vi "Filter VISA COM.vi"(8 "Error In":errorcluster, 11 "Names in":string[](array[string])) -> (0 "Error Out":errorcluster, 2 "Original list":string[](array[string]), 3 "COM only list":string[](array[string]))   [LabVIEW 2018]
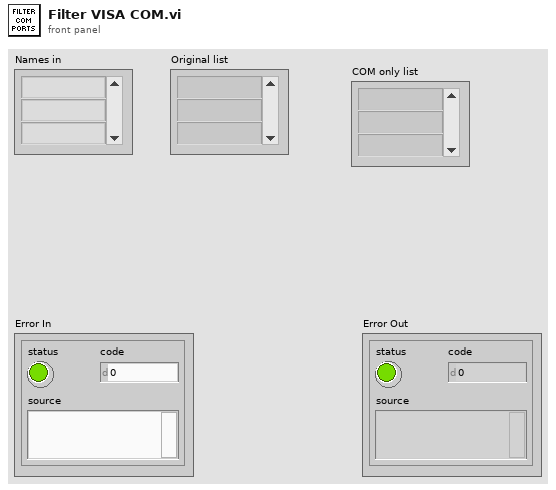
[diagram p1: front panel]
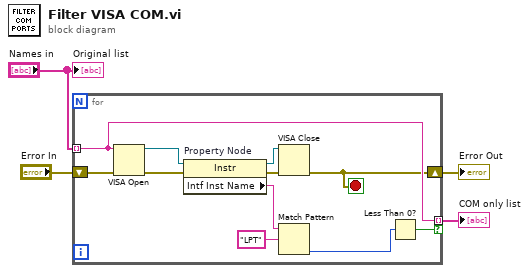
[diagram p0: block diagram]
diagram:
  n1 = for {
    tunnel: "Names in" -> [w9] mode=indexing
    tunnel: [w9] -> w1 mode=indexing if=w7
    shift-right: [w5] -> w3
    shift-left: "Error In" -> [w6]
    stop <- w5 stop-if-true
    n2 = VISA Open(error in (no error)=w6, VISA resource name=w9) -> (VISA resource name=w15:refnum<visa-resource-name>, error out=w14:errorcluster)  [unwired: 3 in]
    n3 = property on="Property Node" class="Instr"(reference=w15, error in=w14) -> (reference out=w13:refnum<visa-resource-name>, error out=w12:errorcluster, "Intf Inst Name"=w11:string)
    n4 = VISA Close(VISA resource name=w13, error in (no error)=w12) -> (error out=w5:errorcluster)
    n5 = Match Pattern(string=w11, regular expression="LPT") -> (offset past match=w8:i32)  [unwired: 1 in, 3 out]
    n6 = Less Than 0?(x=w8) -> (x < 0?=w7:bool)
  }
  "Error Out" <- w3
  "COM only list" <- w1
  "Original list" <- "Names in"
